vi "Target Obsticle Check.vi"(8 "error in (no error)":errorcluster, 11 "DaNI location":dbl[](array[numeric])) -> (0 "error out":errorcluster, 3 "obsticle location":i32[](array[numeric])=[20, 20])   [LabVIEW 2015]
panel:
  out "distance":dbl
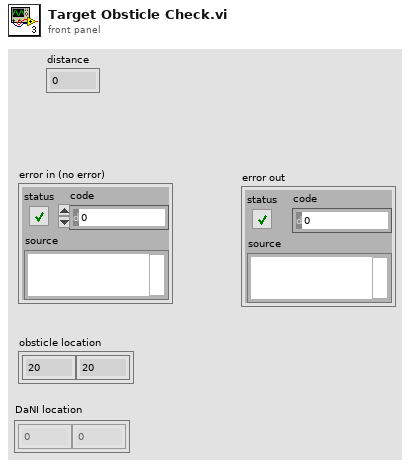
[diagram p1: front panel]
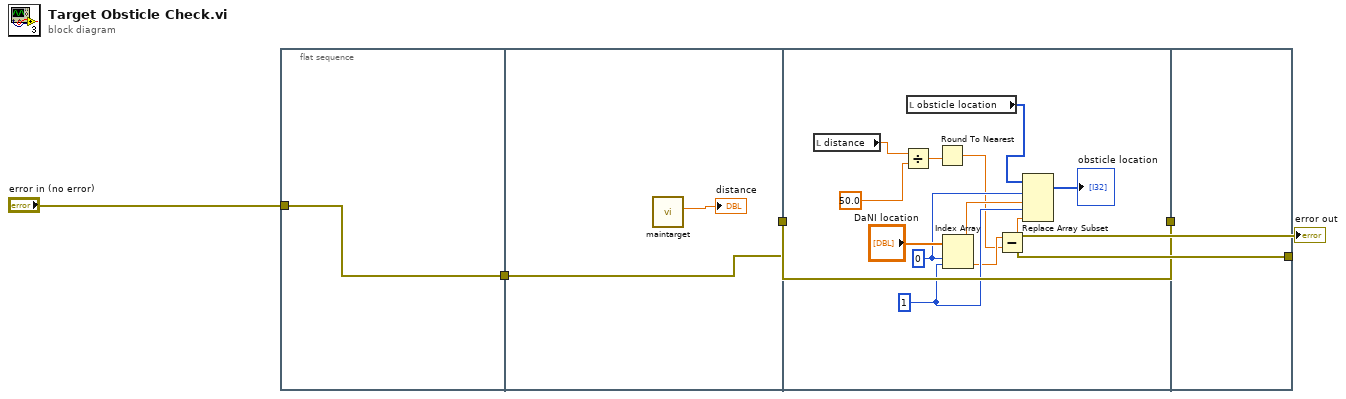
[diagram p0: block diagram]
diagram:
  n1 = flat-sequence {
    tunnel: "error in (no error)" -> [w6]
    tunnel: [w6] -> w4
    tunnel: w4 -> [w7]
    tunnel: [w7] -> w3
    tunnel: w3 -> [w21]
    tunnel: [w21] -> w1
    tunnel: [w22] -> w2
    tunnel: w1 -> [w22]
    frame #0 {
    }
    frame #1 {
      n2 = call "maintarget.vi"() -> ("distance"=→"distance":dbl)  [unwired: 11 in]
    }
    frame #2 {
      w13 = 1
      w14 = 0
      n3 = local read "distance"() -> (w19:dbl)
      n4 = Divide(x=w19, y=50.0) -> (x/y=w18:dbl)
      n5 = local read "obsticle location"() -> (w15:i32[])
      n6 = Round To Nearest(number=w18) -> (nearest integer value=w9:dbl)
      n7 = Index Array(array="DaNI location", index #1=w14, index #2=w13) -> (element #1=w12:dbl, element #2=w10:dbl)
      n8 = Subtract(x=w10, y=w9) -> (x-y=w11:dbl)
      n9 = Replace Array Subset(array=w15, new element #1=w12, index #1=w14, new element #2=w11, index #2=w13) -> (→"obsticle location":i32[])
    }
    frame #3 {
    }
  }
  "error out" <- w2
